vi "Acquisition_pluviometrie_v2.vi"() -> (3 "Numérique":dbl)   [LabVIEW 2017]
doc: "Ce VI fait l'acquisision du pluviomètre (comptage de front)\n\nCopyright | Jixiong Liu & Benoit Mangeard"
uses:
  <vilib>/DAQmx/read.llb/DAQmx Read (Digital Bool 1Line 1Point).vi
  <vilib>/DAQmx/create/channels.llb/DAQmx Create Channel (DI-Digital Input).vi
  <vilib>/DAQmx/miscellaneous.llb/DAQmx Fill In Error Info.vi
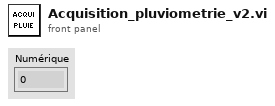
[diagram p1: front panel]
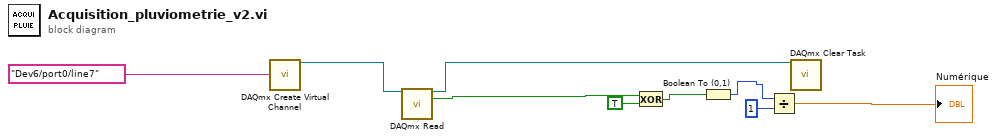
[diagram p0: block diagram]
diagram:
  n1 = call-poly <vilib>:"DAQmx Create Virtual Channel.vi"("lines"=tag "Dev6/port0/line7") -> ("task out"=w2:refnum<k21>)  [unwired: 13 in, 1 out]
  n2 = call-poly <vilib>:"DAQmx Read.vi"("task/channels in"=w2) -> ("task out"=w3:refnum<k21>, "data"=w8:bool)  [unwired: 12 in, 1 out]
  n3 = Exclusive Or(1:TRUE ("y"), 2:w8) -> (0:w5:bool)
  n4 = Boolean To (0,1)(Boolean=w5) -> (0, 1=w6:i16)
  n5 = Divide(x=w6, y=i16 1) -> (x/y=→"Numérique":dbl)
  n6 = call <vilib>:"DAQmx Clear Task.vi"("task in"=w3) -> ()  [unwired: 14 in, 1 out]
